vi "Write Ignore Timestamp.vi"(5 "Ignore Timestamp":bool, 9 "WaveformGraph in":refnum<class "WaveformGraph.lvclass">) -> (3 "WaveformGraph out":refnum<class "WaveformGraph.lvclass">)   [LabVIEW 2014, in "WaveformGraph.lvclass"]
uses:
  WaveformGraph.lvclass
  WaveformGraph.lvclass/WaveformGraph.ctl
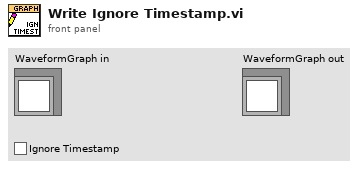
[diagram p1: front panel]
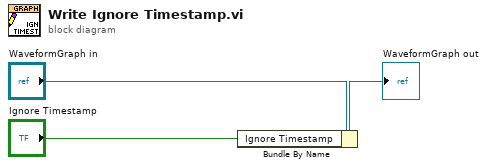
[diagram p0: block diagram]
diagram:
  n1 = Bundle By Name(cluster="WaveformGraph in", "Ignore Timestamp"="Ignore Timestamp") -> (→"WaveformGraph out":refnum<class "WaveformGraph.lvclass">)
